vi "SystemInfo.vi"(7 "LabVIEW Web Service Request":refnum<class "Web Request.lvclass">) -> ()   [LabVIEW 2013]
doc: "SystemInfo provides information about the CPU and memory of the system on which it is run."
uses:
  <vilib>/wsapi/Web Request.lvclass
  <vilib>/NI/TagWebClient/API/tagweb client API.lvlib
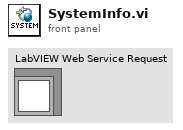
[diagram p1: front panel]
types:
  T1 = typedef "tagweb client API.lvlib/System Info Results.ctl" = cluster{"CPU":dbl, "FreeMemory":dbl, "TotalMemory":dbl, "FreeMemoryPercent":dbl}
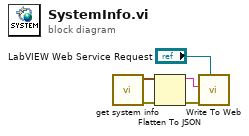
[diagram p0: block diagram]
diagram:
  n1 = call "get system info.vi"() -> ("error out"=w4:errorcluster, "System Info"=w5:T1)  [unwired: 10 in]
  n2 = Flatten To JSON(anything=w5, error in (no error)=w4) -> (JSON string=w1:string, 11:w2:errorcluster)  [unwired: 1 in]
  n3 = call <vilib>:"Write To Web.vi"("Web Request in"="LabVIEW Web Service Request", "error in"=w2, "Response String"=w1) -> ()  [unwired: 9 in]
